vi "Dynamically Call_Settings Info dialog VI.vi"(8 "error in (no error)":errorcluster, 11 "Setting File Type":T1=enum."Configuration Settings") -> (0 "error out":errorcluster)   [LabVIEW 2012]
doc: "SciScan 1.2 160622"
uses:
  Custom Controls/Setting File Types.ctl
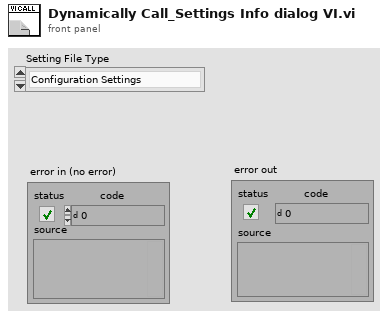
[diagram p1: front panel]
types:
  T1 = typedef "Setting File Types.ctl" = enum16{"2D.Frame.Scan.Settings", "2D.Line.Scan.Settings", "Z.Stack.Settings", "HW Settings", "Configuration Settings", "Unknown Settings", "Fast.Z.Settings"}
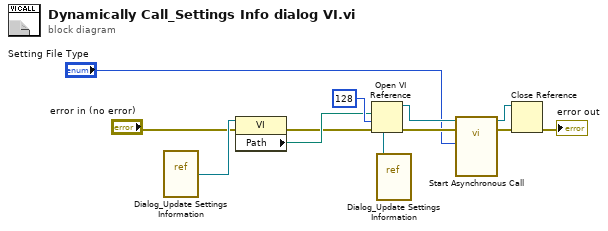
[diagram p0: block diagram]
diagram:
  n1 = vi-ref "Dialog_Update Settings Information.vi"() -> (w8:refnum<vi>)
  n2 = property class="VI"(reference=w8, error in="error in (no error)") -> (error out=w4:errorcluster, "Path"=w7:path)  [unwired: 1 out]
  n3 = vi-ref "Dialog_Update Settings Information.vi"() -> (w12:refnum<vi>)
  n4 = Open VI Reference(type specifier VI Refnum (for type only)=w12, vi path=w7, options=128, error in (no error)=w4) -> (vi reference=w10:refnum<vi>, error out=w9:errorcluster)  [unwired: 2 in]
  n5 = call-by-ref "Start Asynchronous Call"(reference=w10, error in=w9, "Setting File Type"="Setting File Type") -> (reference out=w5:refnum<vi>, error out=w6:errorcluster)  [unwired: 10 in, 1 out]
  n6 = Close Reference(reference=w5, error in (no error)=w6) -> (error out=→"error out":errorcluster)
